vi "setNewItem.vi"(6 "deviceType":T1, 8 "error in (no error)":errorcluster, 9 "dim":i32, 10 "index":i32, 11 "reference in":refnum<class "itemsNotification.lvclass">) -> (0 "error out":errorcluster, 3 "reference out":refnum<class "itemsNotification.lvclass">)   [LabVIEW 2015, in "itemsNotification.lvclass"]
uses:
  itemsNotification.lvclass
  SYS/Devices Controller_llb/deviceType.ctl
  SYS/Devices Controller_llb/Devices Controller.lvclass
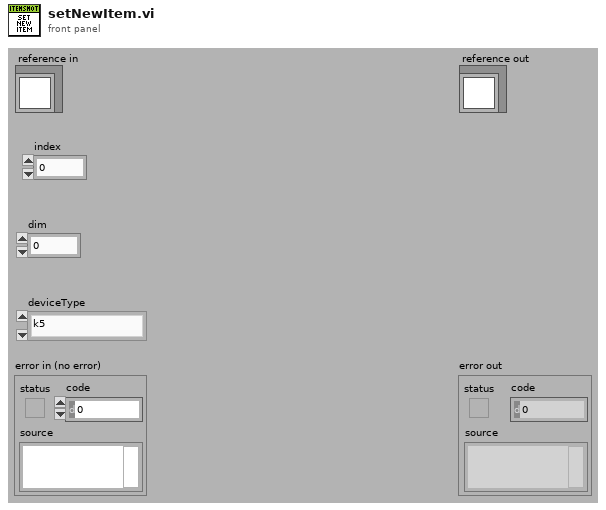
[diagram p1: front panel]
types:
  T1 = typedef "Devices Controller.lvclass/deviceType.ctl" = enum16{"k5", "k4b2", "fitmate", "cpet", "rmr", "bodyBoxPft", "bp", "pp"}
  T2 = typedef "itemsNotification.lvclass/ObjectAttributesRef.ctl" = refnum<data-value>
  T3 = typedef "itemsNotification.lvclass/ObjectAttributes.ctl" = cluster{"MyAttribute":dbl, "details":cluster{"deviceType":T1, "S/N":string, "SW":string, "Description":string, "Account":string, "System's Location":string, "End User":string, "Email":string, "City":string, "LastChange":string, "Service By":string, "Exp Date":string, "FollowUp Sent":string, "FollowUp Accepted":string, "Note":string}}
  T4 = typedef "itemsNotification.lvclass/ClassAttributesRef.ctl" = refnum<data-value>
  T5 = typedef "itemsNotification.lvclass/ClassAttributes.ctl" = cluster{"Dummy":bool, "device_refs":refnum<class "itemsNotification.lvclass">[]}
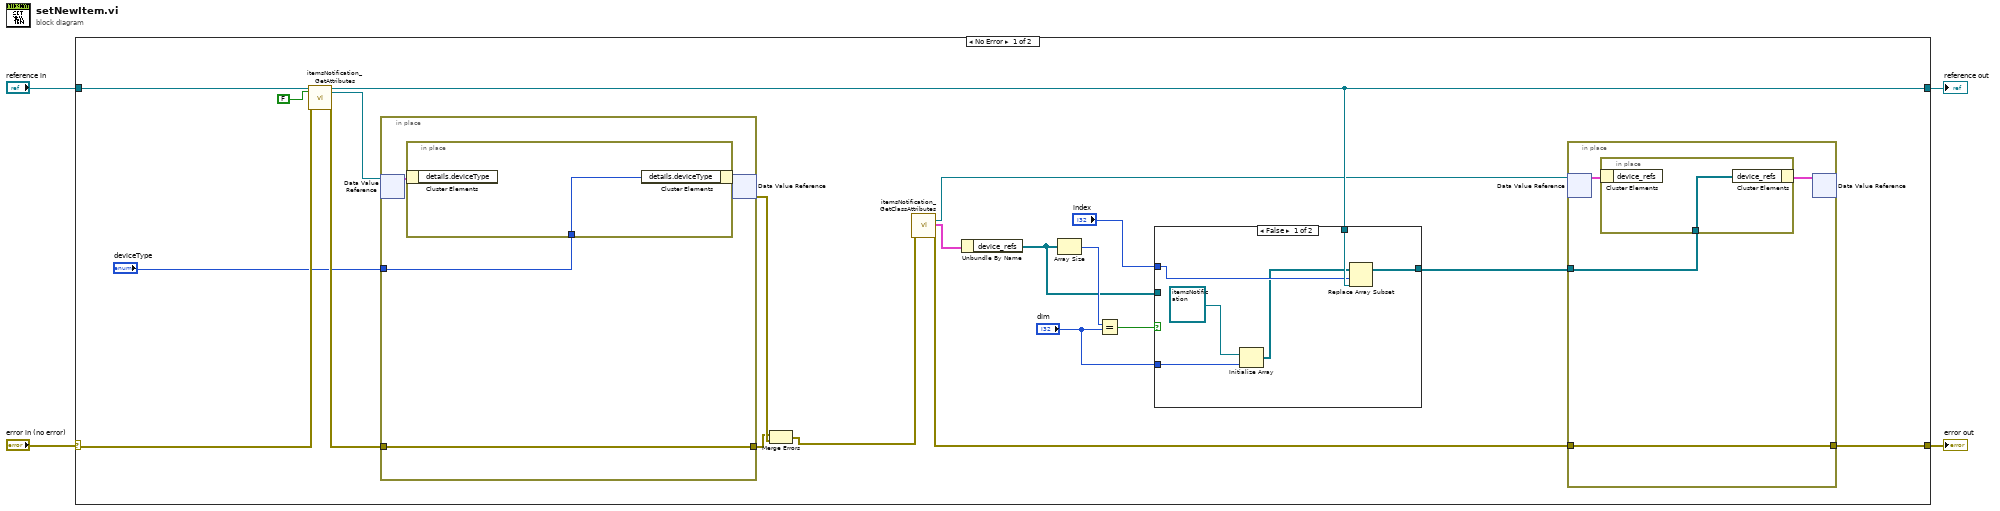
[diagram p0: block diagram]
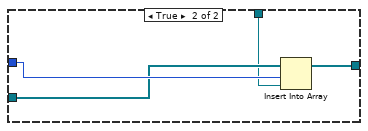
[diagram p2: hidden frame]
diagram:
  n1 = case shown="No Error" "error in (no error)" {
    selector: "error in (no error)" -> [w20 w46]
    tunnel: [w11 w46] -> w3
    tunnel: [w14 w45] -> w1
    tunnel: "reference in" -> [w22 w45]
    frame No Error {
      n2 = call "itemsNotification_GetAttributes.vi"("reference in"=w22, "return data? (T)"=FALSE, "error in (no error)"=w20) -> ("reference out"=w14:refnum<class "itemsNotification.lvclass">, "attributes ref"=w18:T2, "error out"=w19:errorcluster)  [unwired: 13 in, 1 out]
      n3 = in-place {
        in-place-border: w19 -> [w41]
        in-place-border: [w41] -> w23
        in-place-border: "deviceType" -> [w40]
        n4 = in-place-dvr #1(w18) -> (w42:T3)  [unwired: 1 out]
        n5 = in-place {
          in-place-border: w40 -> [w44]
          n6 = in-place-cluster #2(w42) -> ()  [unwired: 1 out]
          n7 = in-place-cluster #2("details.deviceType"=w44) -> (w43:T3)
        }
        n8 = in-place-dvr #1(w43) -> (w24:errorcluster)  [unwired: 1 out]
      }
      n9 = Merge Errors(w23, w24) -> (w8:errorcluster)
      n10 = call "itemsNotification_GetClassAttributes.vi"("error in (no error)"=w8) -> ("class attributes ref"=w10:T4, "class attributes"=w17:T5, "error out"=w12:errorcluster)  [unwired: 15 in, 1 out]
      n11 = Unbundle By Name(w17) -> ("device_refs"=w13:refnum<class "itemsNotification.lvclass">[])
      n12 = Array Size(array=w13) -> (size(s)=w16:i32)
      n13 = Equal?(x=w16, y="dim") -> (x = y?=w15:bool)
      n14 = case shown="False" w15 {
        tunnel: "index" -> [w34 w39]
        tunnel: w14 -> [w35 w36]
        tunnel: w13 -> [_ w38]
        tunnel: [w32 w37] -> w9
        tunnel: "dim" -> [w30 _]
        frame False {
          n15 = Initialize Array(refnum<class "itemsNotification.lvclass"> refnum ("device.lvclass"), w30) -> (w33:refnum<class "itemsNotification.lvclass">[])
          n16 = Replace Array Subset(array=w33, new element=w35, index=w34) -> (w32:refnum<class "itemsNotification.lvclass">[])
        }
        frame True {
          n17 = Insert Into Array(array=w38, index=w39, new element=w36) -> (w37:refnum<class "itemsNotification.lvclass">[])
        }
      }
      n18 = in-place {
        in-place-border: w12 -> [w26]
        in-place-border: [w26] -> w11
        in-place-border: w9 -> [w25]
        n19 = in-place-dvr #3(w10) -> (w27:T5)  [unwired: 1 out]
        n20 = in-place {
          in-place-border: w25 -> [w29]
          n21 = in-place-cluster #4(w27) -> ()  [unwired: 1 out]
          n22 = in-place-cluster #4("device_refs"=w29) -> (w28:T5)
        }
        n23 = in-place-dvr #3(w28) -> ()  [unwired: 2 out]
      }
    }
    frame Error {
    }
  }
  "error out" <- w3
  "reference out" <- w1
